vi "check x mirror speed.vi"() -> (3 "mirror speed valid":bool)   [LabVIEW 2012]
doc: "SciScan 1.2 160622"
uses:
  GFG/GFGnumericGet.vi
  GFG/GFGbooleanGet.vi
  GFG/GFGfpRefGet.vi
  GFG/GFG library.lvlib
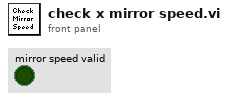
[diagram p1: front panel]
types:
  T1 = cluster{"Boolean":bool, "Numeric":dbl, "Numeric":dbl}
  T2 = cluster{"Boolean Value OUT":bool, "Numeric":dbl, "Numeric":dbl}
  T3 = enum8{"Enabled", "Disabled", "Disabled and Grayed Out"}
  T4 = cluster{"WaveformChartRef":refnum<vi>, "DigitalRef":refnum<vi>, "ArrayRef":refnum<vi>, "TabControlRef":refnum<vi>, "EnumRef":refnum<vi>, "RingRef":refnum<vi>, "BooleanRef":refnum<vi>, "KnobRef":refnum<vi>, "SlideRef":refnum<vi>, "PathRef":refnum<vi>, "StringRef":refnum<vi>, "ComboBox":refnum<vi>, "WaveformGraphRef":refnum<vi>}
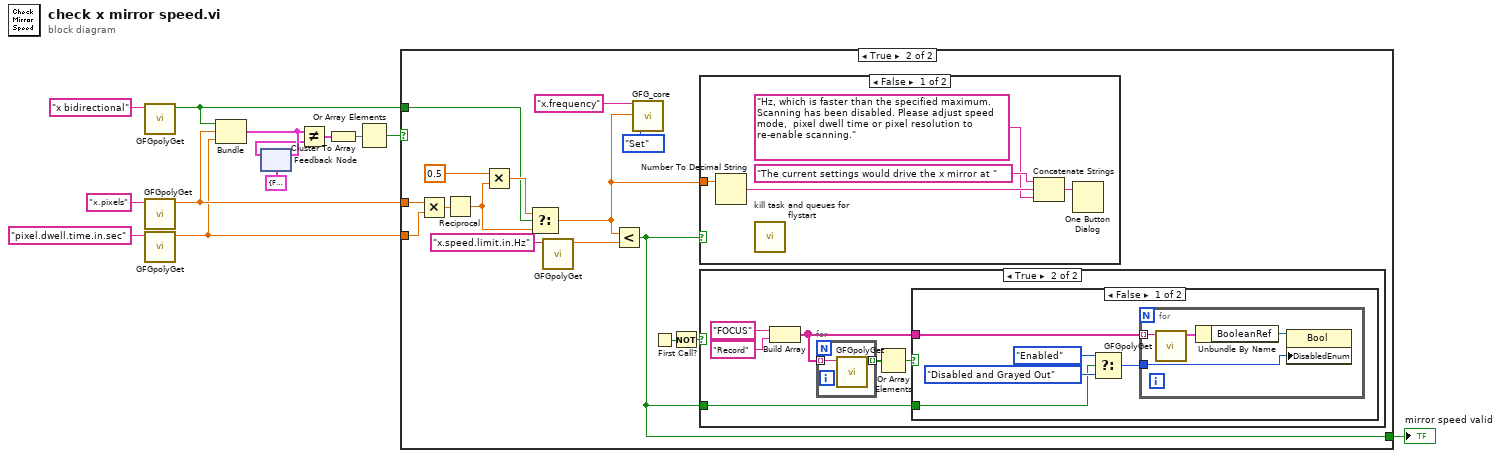
[diagram p0: block diagram]
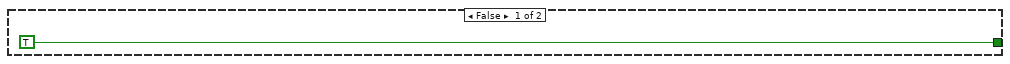
[diagram p2: hidden frame]
diagram:
  n1 = call-poly "GFGpolyGet.vi"("Variable Name in"="x bidirectional") -> ("Boolean Value OUT"=w10:bool)  [unwired: 9 in, 1 out]
  n2 = call-poly "GFGpolyGet.vi"("Variable Name in"="x.pixels") -> ("Numeric"=w9:dbl)  [unwired: 8 in, 2 out]
  n3 = call-poly "GFGpolyGet.vi"("Variable Name in"="pixel.dwell.time.in.sec") -> ("Numeric"=w8:dbl)  [unwired: 8 in, 2 out]
  n4 = Bundle("Boolean Value OUT"=w10, "Numeric"=w9, "Numeric"=w8) -> (w6:T2)  [unwired: 1 in]
  n5 = feedback #1(T1 {"Boolean"=FALSE, "Numeric"=0.0, "Numeric"=0.0}) -> (w5:T1)
  n6 = feedback-in #1(w6) -> ()
  n7 = Not Equal?(x=w6, y=w5) -> (x != y?=w4:cluster{bool, "Numeric":bool, "Numeric":bool})
  n8 = Cluster To Array(cluster=w4) -> (array=w2:bool[])
  n9 = Or Array Elements(Boolean array=w2) -> (logical OR=w3:bool)
  n10 = case shown="True" w3 {
    tunnel: w10 -> [_ w26]
    tunnel: w9 -> [_ w24]
    tunnel: w8 -> [_ w23]
    tunnel: [TRUE w22] -> w1
    frame False {
    }
    frame True {
      n11 = Multiply(x=w24, y=w23) -> (x*y=w25:dbl)
      n12 = Reciprocal(x=w25) -> (1/x=w16:dbl)
      n13 = Multiply(x=0.5 ("y"), y=w16) -> (x*y=w27:dbl)
      n14 = Select(t=w27, s=w26, f=w16) -> (s? t:f=w17:dbl)
      n15 = call-poly "GFGpolyGet.vi"("Variable Name in"="x.speed.limit.in.Hz") -> ("Numeric"=w29:dbl)  [unwired: 8 in, 2 out]
      n16 = Less?(x=w17, y=w29) -> (x < y?=w22:bool)
      n17 = call "GFG_core.vi"("Variable Name in"="x.frequency", "Variant in"=w17, "Action"=enum16{"Init", "Set", "Get"}."Set") -> ()  [unwired: 10 in, 7 out]
      n18 = First Call?() -> (First Call?: T/F=w21:bool)
      n19 = Not(x=w21) -> (.not. x?=w20:bool)
      n20 = case shown="False" w22 {
        tunnel: w17 -> [w51 _]
        frame False {
          n21 = Number To Decimal String(number=w51) -> (decimal integer string=w49:string)  [unwired: 1 in]
          n22 = call "kill task and queues for flystart.vi"() -> ()  [unwired: 12 in]
          n23 = Concatenate Strings("The current settings would drive the x mirror at " ("message"), w49, "Hz, which is faster than the specified maximum. Scanning has been disabled. Please adjust speed mode,  pixel dwell time or pixel resolution to re-enable scanning." ("string")) -> (w47:string)
          n24 = One Button Dialog(message=w47) -> ()  [unwired: 1 in, 1 out]
        }
        frame True {
        }
      }
      n25 = case shown="True" w20 {
        tunnel: w22 -> [_ w33]
        frame False {
        }
        frame True {
          n26 = Build Array("FOCUS" ("Variable Name in"), "Record" ("element")) -> (w32:string[])
          n27 = for {
            tunnel: w32 -> [w46] mode=indexing
            tunnel: [w45] -> w31 mode=indexing
            n28 = call-poly "GFGpolyGet.vi"("Variable Name in"=w46) -> ("Boolean Value OUT"=w45:bool)  [unwired: 9 in, 1 out]
          }
          n29 = Or Array Elements(Boolean array=w31) -> (logical OR=w30:bool)
          n30 = case shown="False" w30 {
            tunnel: w33 -> [w37 _]
            tunnel: w32 -> [w36 _]
            frame False {
              n31 = Select(t=T3."Enabled" ("Disabled"), s=w37, f=T3."Disabled and Grayed Out" ("Disabled")) -> (s? t:f=w38:T3)
              n32 = for {
                tunnel: w36 -> [w42] mode=indexing
                tunnel: w38 -> [w41]
                n33 = call-poly "GFGpolyGet.vi"("Variable Name in"=w42) -> ("output cluster"=w44:T4)  [unwired: 9 in, 1 out]
                n34 = Unbundle By Name(w44) -> ("BooleanRef"=w43:refnum<vi>)
                n35 = property class="Bool"(reference=w43, "DisabledEnum"=w41) -> ()  [unwired: 1 in, 2 out]
              }
            }
            frame True {
            }
          }
        }
      }
    }
  }
  "mirror speed valid" <- w1
